vi "CALCULADORA1.vi"() -> ()   [LabVIEW 2020]
panel:
  out "GRAFICO":dbl(graph)
  in  "?":bool
  out "RESULTADO":dbl
  in  "VALOR 2":dbl
  in  "VALOR 1":dbl
  in  "OPCIONES":T1(ring)
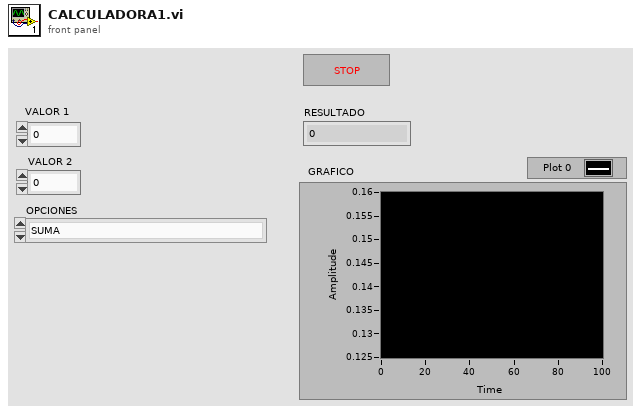
[diagram p1: front panel]
types:
  T1 = enum16{"SUMA", "RESTA", "MULTIPLICACION ", "DIVISION ", "RAIZ CUADRADA", "EXPONENCIAL", "CONV. °GRAD A RAD", "FUNCIONES TRIGONOMETRICAS- SENO", "COSENO ", "TANGENTE"}
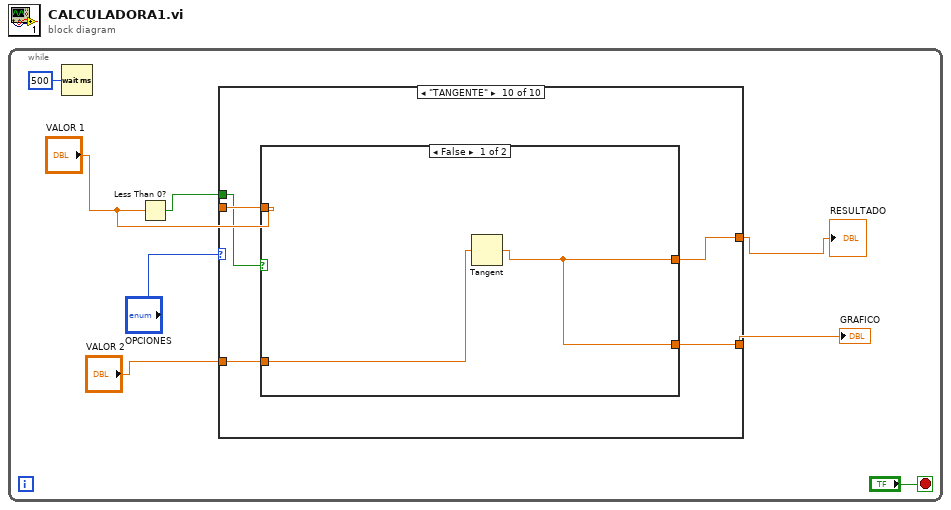
[diagram p0: block diagram]
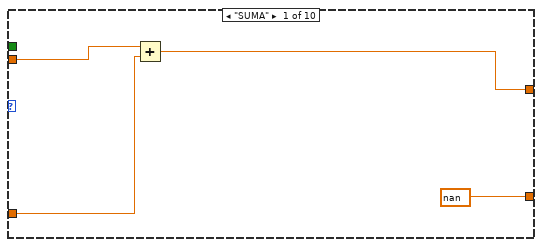
[diagram p2: hidden frame]
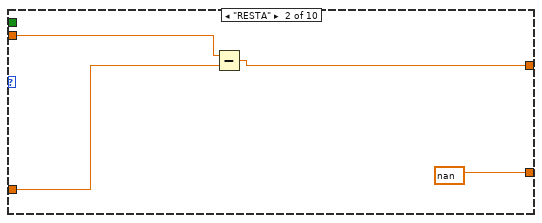
[diagram p3: hidden frame]
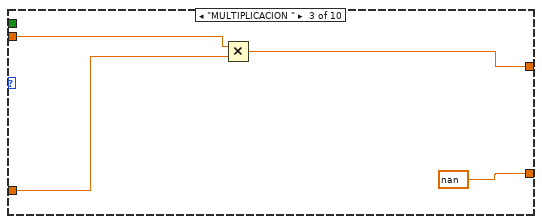
[diagram p4: hidden frame]
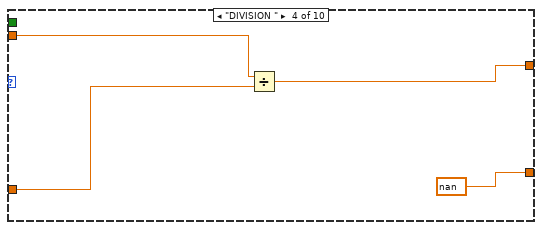
[diagram p5: hidden frame]
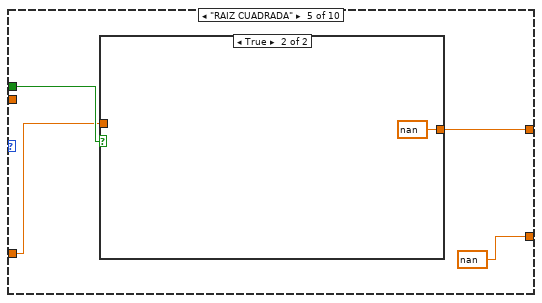
[diagram p6: hidden frame]
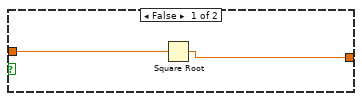
[diagram p7: hidden frame]
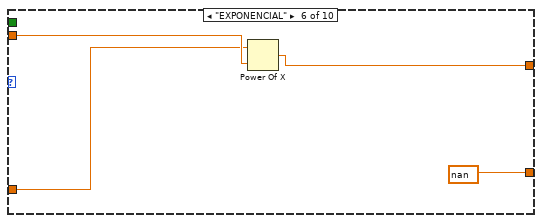
[diagram p8: hidden frame]
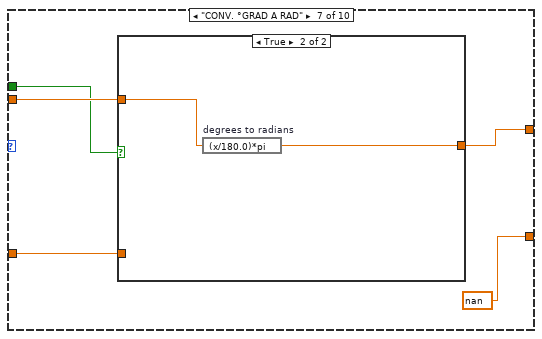
[diagram p9: hidden frame]
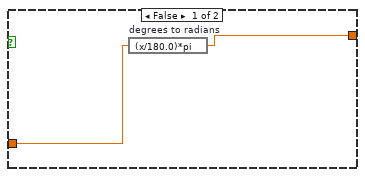
[diagram p10: hidden frame]
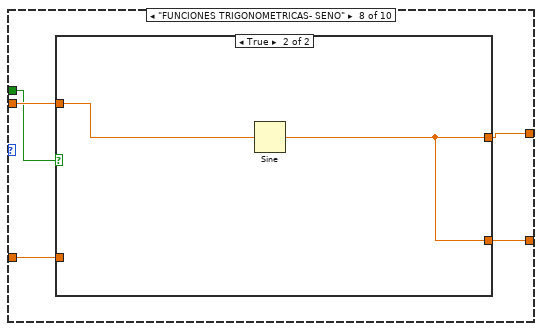
[diagram p11: hidden frame]
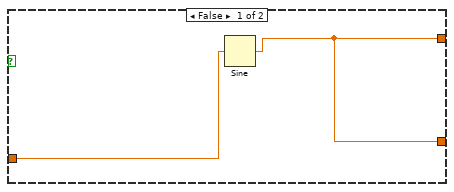
[diagram p12: hidden frame]
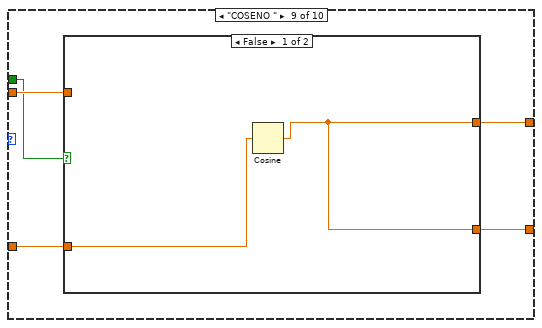
[diagram p13: hidden frame]
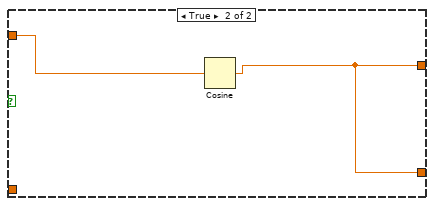
[diagram p14: hidden frame]
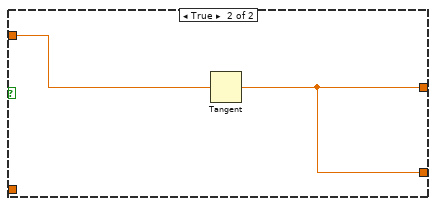
[diagram p15: hidden frame]
diagram:
  n1 = while {
    stop <- "?" stop-if-true
    n2 = Wait (ms)(milliseconds to wait=u32 500) -> ()  [unwired: 1 out]
    n3 = Less Than 0?(x="VALOR 1") -> (x < 0?=w7:bool)
    n4 = case shown="\"TANGENTE\"" "OPCIONES" {
      tunnel: w7 -> [_ _ _ _ w26 _ w36 w45 w56 w65]
      tunnel: "VALOR 2" -> [w12 w16 w20 w24 w25 w33 w38 w46 w54 w63]
      tunnel: [w10 w14 w18 w22 w28 w35 w39 w48 w57 w66] -> w3
      tunnel: "VALOR 1" -> [w11 w15 w19 w23 _ w34 w40 w49 w58 w67]
      tunnel: [nan nan nan nan nan nan nan w47 w55 w64] -> w2
      frame "SUMA" {
        n5 = Add(x=w11, y=w12) -> (x+y=w10:dbl)
      }
      frame "RESTA" {
        n6 = Subtract(x=w15, y=w16) -> (x-y=w14:dbl)
      }
      frame "MULTIPLICACION " {
        n7 = Multiply(x=w19, y=w20) -> (x*y=w18:dbl)
      }
      frame "DIVISION " {
        n8 = Divide(x=w23, y=w24) -> (x/y=w22:dbl)
      }
      frame "RAIZ CUADRADA" {
        n9 = case shown="True" w26 {
          tunnel: [w30 nan] -> w28
          tunnel: w25 -> [w29 _]
          frame False {
            n10 = Square Root(x=w29) -> (sqrt(x)=w30:dbl)
          }
          frame True {
          }
        }
      }
      frame "EXPONENCIAL" {
        n11 = Power Of X(1:w34, 2:w33) -> (0:w35:dbl)
      }
      frame "CONV. °GRAD A RAD" {
        n12 = case shown="True" w36 {
          tunnel: w40 -> [_ w44]
          tunnel: [w41 w43] -> w39
          tunnel: w38 -> [w42 _]
          frame False {
            n13 = expression code="(x/180.0)*pi" "degrees to radians"(w42) -> (w41:dbl)
          }
          frame True {
            n14 = expression code="(x/180.0)*pi" "degrees to radians"(w44) -> (w43:dbl)
          }
        }
      }
      frame "FUNCIONES TRIGONOMETRICAS- SENO" {
        n15 = case shown="True" w45 {
          tunnel: w49 -> [_ w53]
          tunnel: [w50 w52] -> w48
          tunnel: [w50 w52] -> w47
          tunnel: w46 -> [w51 _]
          frame False {
            n16 = Sine(x=w51) -> (sin(x)=w50:dbl)
          }
          frame True {
            n17 = Sine(x=w53) -> (sin(x)=w52:dbl)
          }
        }
      }
      frame "COSENO " {
        n18 = case shown="False" w56 {
          tunnel: w58 -> [_ w62]
          tunnel: [w59 w61] -> w57
          tunnel: [w59 w61] -> w55
          tunnel: w54 -> [w60 _]
          frame False {
            n19 = Cosine(x=w60) -> (cos(x)=w59:dbl)
          }
          frame True {
            n20 = Cosine(x=w62) -> (cos(x)=w61:dbl)
          }
        }
      }
      frame "TANGENTE" {
        n21 = case shown="False" w65 {
          tunnel: w67 -> [_ w71]
          tunnel: [w69 w70] -> w66
          tunnel: [w69 w70] -> w64
          tunnel: w63 -> [w68 _]
          frame False {
            n22 = Tangent(1:w68) -> (0:w69:dbl)
          }
          frame True {
            n23 = Tangent(1:w71) -> (0:w70:dbl)
          }
        }
      }
    }
    "RESULTADO" <- w3
    "GRAFICO" <- w2
  }
